vi "uPublisher BatchPublish.vi"(8 "error in (no error)":errorcluster, 10 "uMsgs":refnum<class "uMsg.lvclass">[](array[class]), 11 "uClient_Publisher in":refnum<class "uClient_Publisher.lvclass">) -> (0 "error out":errorcluster, 3 "uClient_Publisher out":refnum<class "uClient_Publisher.lvclass">)   [LabVIEW 2021, in "uFramework.lvlib" / "uClient_Publisher.lvclass"]
doc: "Publish a batch of event to the broker in performance optimized manner."
uses:
  uClient_Publisher.lvclass
  uClient_Publisher.lvclass/uClient_Publisher.ctl
  Bin/uData.lvlibp/uData.lvclass
  uMsg/uMsg.lvclass
  Bin/uStringManipulation.lvlibp/uStringManipulation.lvclass
  U:/Projects/uFramework/Src/uFramework/uClient/uClient.lvclass
  U:/Projects/uFramework/Src/uFramework/uClient_Publisher/uClient_Publisher.lvclass
  U:/Projects/uFramework/Src/uFramework/uTransport/uTransport.lvclass
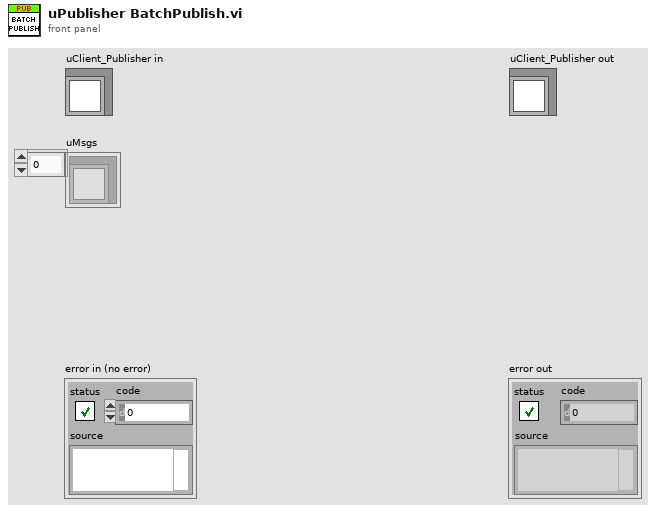
[diagram p1: front panel]
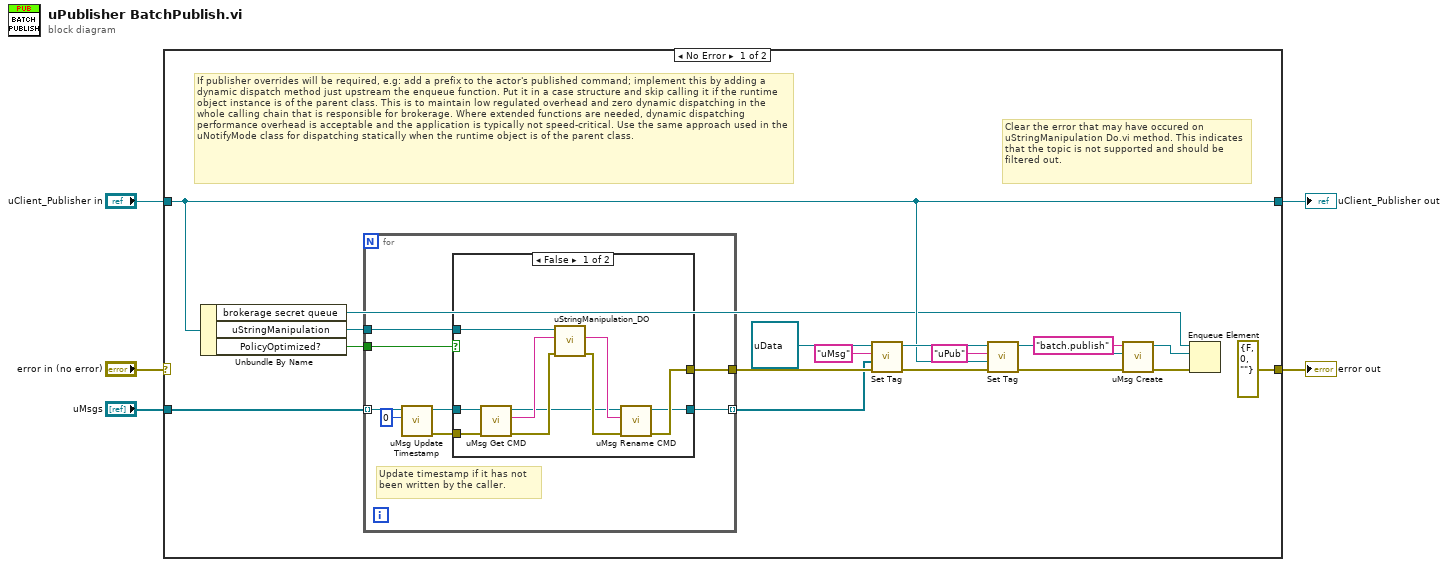
[diagram p0: block diagram]
diagram:
  n1 = case shown="No Error" "error in (no error)" {
    selector: "error in (no error)" -> [_ w44]
    tunnel: [errorcluster {"status"=FALSE, "code"=0, "source"=""} ("error IO") w44] -> w5
    tunnel: "uClient_Publisher in" -> [w12 w45]
    tunnel: "uMsgs" -> [w7 _]
    tunnel: [w12 w45] -> w2
    frame No Error {
      # "Clear the error that may have occured on uStringManipulation Do.vi method. This indicates that the topic is not supported and should be filtered out."
      # "If publisher overrides will be required, e.g: add a prefix to the actor's published command; implement this by adding a dynamic dispatch method just upstream the enqueue function. Put it in a case structure and skip calling it if the runtime object instance is of the parent class. This is to maintain low regulated overhead and zero dynamic dispatching in the whole calling chain that is responsible for brokerage. Where extended functions are needed, dynamic dispatching performance overhead is acceptable and the application is typically not speed-critical. Use the same approach used in the uNotifyMode class for dispatching statically when the runtime object is of the parent class."
      n2 = Unbundle By Name(w12) -> ("brokerage secret queue"=w6:refnum<queue>, "uStringManipulation"=w13:refnum<class "uStringManipulation.lvclass">, "PolicyOptimized?"=w8:bool)
      n3 = for {
        tunnel: [w31] -> w15
        tunnel: [w30] -> w14 mode=indexing
        tunnel: w13 -> [w29]
        tunnel: w8 -> [w28]
        tunnel: w7 -> [w25] mode=indexing
        # "Update timestamp if it has not been written by the caller."
        n4 = call "uMsg Update Timestamp.vi"("Timestamp"=u32 0, "uMsg in"=w25) -> ("error out"=w24:errorcluster, "uMsg out"=w26:refnum<class "uMsg.lvclass">)  [unwired: 8 in]
        n5 = case shown="False" w28 {
          tunnel: w29 -> [w41 _]
          tunnel: [w40 w43] -> w31
          tunnel: w26 -> [w37 w42]
          tunnel: [w38 w42] -> w30
          tunnel: w24 -> [w33 w43]
          frame False {
            n6 = call "uMsg Get CMD.vi"("error in (no error)"=w33, "uMsg in"=w37) -> ("error out"=w36:errorcluster, "CMD"=w34:string, "uMsg out"=w32:refnum<class "uMsg.lvclass">)  [unwired: 7 in]
            n7 = call-dynamic "uStringManipulation_DO.vi"("error in (no error)"=w36, "String in"=w34, "uStringManipulation in"=w41) -> ("error out"=w35:errorcluster, "String"=w39:string)  [unwired: 6 in, 1 out]
            n8 = call "uMsg Rename CMD.vi"("error in (no error)"=w35, "New CMD"=w39, "uMsg in"=w32) -> ("error out"=w40:errorcluster, "uMsg out"=w38:refnum<class "uMsg.lvclass">)  [unwired: 7 in]
          }
          frame True {
            # "Avoid the unnecessary dynamic dispatch uStringManipulation method's overhead  if there is no translation provided."
          }
        }
      }
      n9 = call "Set Tag.vi"("error in (no error)"=w15, "Variant"=w14, "tag (case insensitive)"="uMsg", "uData in"=refnum<class "uData.lvclass"> refnum) -> ("error out"=w21:errorcluster, "uData out"=w19:refnum<class "uData.lvclass">)  [unwired: 5 in, 1 out]
      n10 = call "Set Tag.vi"("error in (no error)"=w21, "Variant"=w12, "tag (case insensitive)"="uPub", "uData in"=w19) -> ("error out"=w23:errorcluster, "uData out"=w16:refnum<class "uData.lvclass">)  [unwired: 5 in, 1 out]
      n11 = call "uMsg Create.vi"("error in (no error)"=w23, "Payload"=w16, "CMD"="batch.publish") -> ("error out"=w9:errorcluster, "uMsg out"=w10:refnum<class "uMsg.lvclass">)  [unwired: 7 in]
      n12 = Enqueue Element(queue=w6, element=w10, error in (no error)=w9) -> ()  [unwired: 1 in, 3 out]
    }
    frame Error {
    }
  }
  "error out" <- w5
  "uClient_Publisher out" <- w2
